vi "Switch Making Connection.vi"(8 "error in (no error)":errorcluster, 9 "Second Connection":cluster{"channel 3":string, "channel 4":string}={"channel 3"="r1", "channel 4"="c1"}, 10 "First Connection":cluster{"channel 1":string, "channel 2":string}={"channel 1"="r0", "channel 2"="c0"}, 11 "PXIe 2737 in":refnum<class "PXIe 2737.lvclass">) -> (0 "error out":errorcluster, 3 "PXIe 2737 out":refnum<class "PXIe 2737.lvclass">)   [LabVIEW 2016, in "S-Matrix.lvlib" / "PXIe 2737.lvclass"]
uses:
  PXIe 2737.lvclass
  PXIe 2737.lvclass/PXIe 2737.ctl
  <instrlib>/niSwitch/niSwitch.llb/niSwitch Connect Channels (Single).vi
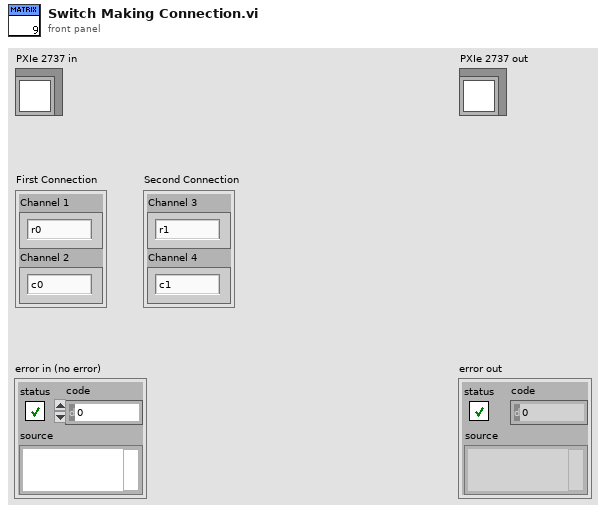
[diagram p1: front panel]
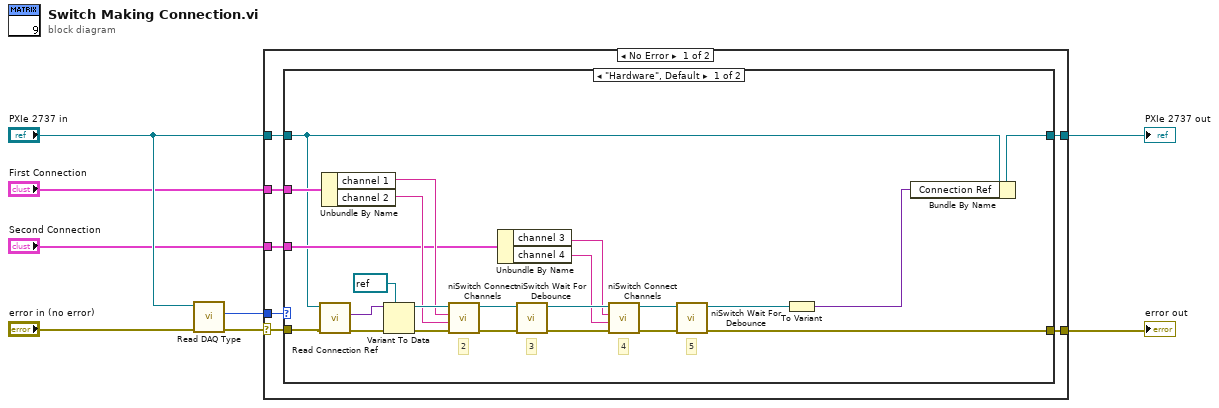
[diagram p0: block diagram]
diagram:
  n1 = call-dynamic "Read DAQ Type.vi"("error in (no error)"="error in (no error)", "PXIe 2737 in"="PXIe 2737 in") -> ("error out"=w7:errorcluster, "DAQ Type"=w5:enum16{"Hardware", "Simulation"})  [unwired: 7 in, 1 out]
  n2 = case shown="No Error" w7 {
    selector: w7 -> [w15 w41]
    tunnel: "PXIe 2737 in" -> [w13 w42]
    tunnel: w5 -> [w14 _]
    tunnel: "First Connection" -> [w12 _]
    tunnel: "Second Connection" -> [w11 _]
    tunnel: [w10 w42] -> w1
    tunnel: [w9 w41] -> w2
    frame No Error {
      n3 = case shown="\"Hardware\", Default" w14 {
        tunnel: w15 -> [w38 w39]
        tunnel: w13 -> [w20 w40]
        tunnel: w12 -> [w31 _]
        tunnel: w11 -> [w23 _]
        tunnel: [w18 w40] -> w10
        tunnel: [w19 w39] -> w9
        frame "Hardware", Default {
          # "4"
          # "5"
          # "3"
          # "2"
          n4 = call-dynamic "Read Connection Ref.vi"("error in (no error)"=w38, "PXIe 2737 in"=w20) -> ("error out"=w30:errorcluster, "Connection Ref"=w28:variant)  [unwired: 7 in, 1 out]
          n5 = Unbundle By Name(w31) -> ("channel 1"=w25:string, "channel 2"=w24:string)
          n6 = Variant To Data(error in=w30, type=refnum<k15> refnum ("instrument handle"), Variant=w28) -> (data=w26:refnum<k15>, error out=w29:errorcluster)
          n7 = call-poly <instrlib>:"niSwitch Connect Channels.vi"("error in (no error)"=w29, "channel 2"=w24, "channel 1"=w25, "instrument handle"=w26) -> ("error out"=w37:errorcluster, "instrument handle out"=w36:refnum<k15>)  [unwired: 6 in]
          n8 = Unbundle By Name(w23) -> ("channel 3"=w22:string, "channel 4"=w21:string)
          n9 = call <instrlib>:"niSwitch Wait For Debounce.vi"("error in (no error)"=w37, "instrument handle"=w36) -> ("error out"=w32:errorcluster, "instrument handle out"=w33:refnum<k15>)  [unwired: 1 in, 7 out]
          n10 = call-poly <instrlib>:"niSwitch Connect Channels.vi"("error in (no error)"=w32, "channel 2"=w21, "channel 1"=w22, "instrument handle"=w33) -> ("error out"=w34:errorcluster, "instrument handle out"=w35:refnum<k15>)  [unwired: 6 in]
          n11 = call <instrlib>:"niSwitch Wait For Debounce.vi"("error in (no error)"=w34, "instrument handle"=w35) -> ("error out"=w19:errorcluster, "instrument handle out"=w17:refnum<k15>)  [unwired: 1 in, 7 out]
          n12 = To Variant(anything=w17) -> (Variant=w16:variant)
          n13 = Bundle By Name(cluster=w20, "Connection Ref"=w16) -> (w18:refnum<class "PXIe 2737.lvclass">)
        }
        frame "Simulation" {
        }
      }
    }
    frame Error {
    }
  }
  "error out" <- w2
  "PXIe 2737 out" <- w1
